vi "Read Value2.vi"(11 "Effect Interface in":refnum<class "Effect Interface.lvclass">) -> (2 "Value Cluster":T1, 3 "Effect Interface out":refnum<class "Effect Interface.lvclass">)   [LabVIEW 2019, in "Effect Interface.lvlib" / "Effect Interface.lvclass"]
uses:
  Effect Interface.lvclass
  Libraries/Audio Processing/Value Cluster.ctl
  Libraries/Audio Processing/Value Properties.ctl
  Effect Interface.lvclass/Effect Interface.ctl
  Libraries/Audio Processing/Audio Processing.lvlib
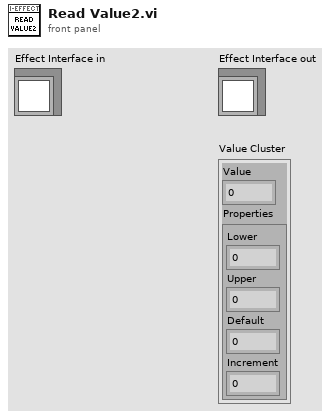
[diagram p1: front panel]
types:
  T1 = typedef "Audio Processing.lvlib/Value Cluster.ctl" = cluster{"Value":dbl, "Properties":T2}
  T2 = typedef "Audio Processing.lvlib/Value Properties.ctl" = cluster{"Lower":dbl, "Upper":dbl, "Default":dbl, "Increment":dbl}
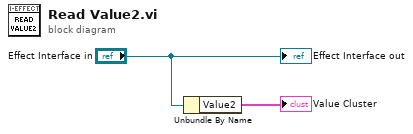
[diagram p0: block diagram]
diagram:
  n1 = Unbundle By Name("Effect Interface in") -> ("Value2"=→"Value Cluster":T1)
  "Effect Interface out" <- "Effect Interface in"
